vi "Target.vi"() -> ()   [LabVIEW 2018]
uses:
  <vilib>/Platform/TimedLoop/XDataNode/timing_clust.ctl
  <vilib>/Platform/TimedLoop/XDataNode/nitl_modes.ctl
  <vilib>/Platform/TimedLoop/XDataNode/wakeup.ctl
  <vilib>/rvi/eio/common/nirviEmuTemplateMethod_errors.vi
  <vilib>/rvi/Emulation/niFpgaSctlEmulationGetInTimedLoop.vi
  <vilib>/rvi/Emulation/niFpgaEmulationReportErrorSimple.vi
  <vilib>/rvi/Emulation/niFpgaGetClockAttributes.vi
  <vilib>/rvi/Emulation/niFpgaCriticalErrorInLSC.vi
  <vilib>/rvi/Emulation/niFpgaProcessEmulError.vi
  <vilib>/rvi/Memory/Memory_Emulation/niFpgaMemoryFastEmulationDramWriteAndRequestData.vi
  <vilib>/rvi/Memory/Memory_Emulation/niFpgaMemoryEmulationDramWriteAndRequestData.vi
  <vilib>/rvi/DataTransferAndStorage/Container/Common/niFpgaContainerGetUniqueNameForEmu.vi
  <vilib>/rvi/Memory/Memory_Emulation/niFpgaMemoryEmulationDramWriteAndRequestDataApplyByteEnables.vi
  <vilib>/rvi/interface/RandomDataEmulation/niFpgaRandomDataHandleErrors.vi
  <vilib>/eio/EIONode/EIONode.xnode
  <vilib>/Platform/TimedLoop/XDataNode/XDataNode.xnode
  <vilib>/rvi/DataTransferAndStorage/Container/XNode/niFpgaContainer.xnode
  <vilib>/rvi/Memory/Memory_Emulation/niFpgaMemoryEmulationDramRetrieveData.vi
  <vilib>/rvi/interface/RandomDataEmulation/nirviRandomDataFpgaReadWriteTemplate.vi
  <vilib>/Platform/TimedLoop/XDataNode/XDNodeRunTimeDep.lvlib
panel:
  in  "46":u8=46
  in  "94":u8=94
  in  "39":u8=39
  in  "95":u8=95
  in  "93":u8=93
  in  "38":u8=38
  in  "R35":u8=35
  in  "92":u8=92
  in  "75":u8=75
  in  "74":u8=74
  in  "56":u8=56
  in  "W35":u8=35
  in  "W75":u8=75
  in  "W1":u8=1
  in  "25":u8=25
  out "Read":bool[](array[boolean])
  in  "Write":bool[](array[boolean])=[FALSE, FALSE, FALSE, FALSE, FALSE, FALSE, FALSE, FALSE, FALSE, FALSE, FALSE, FALSE, FALSE, FALSE, FALSE, FALSE, FALSE, FALSE, FALSE, FALSE, FALSE, FALSE, FALSE, FALSE, FALSE, FALSE, FALSE, FALSE, FALSE, FALSE, FALSE, FALSE, FALSE, FALSE, FALSE]
  in  "Чтение_48":u8=48
  in  "Запись_38":u8=38
  in  "Запись(T)/Чтение(F)":bool
  in  "50":u8=50
  in  "EXPOSURE":bool
  in  "RESET_BAR":bool
  in  "STANDBY":bool
  in  "Кадр на ПК":bool
  in  "Нач_адр":u32
  in  "Кон_адр":u32=120320
  out "Записали FIFO":bool
  in  "Кадр в память":bool
  out "Записали адресов":u32
  in  "Направление бит":bool
  in  "360960":u32=360960
  in  "Стоп":bool
  in  "Регистр":bool
  # "Используется для записи и перед чтением"
  # "D0"
  # "D7"
  # "\"0\""
  # "D8"
  # "D15"
  # "\"0\""
  # "R0"
  # "R7"
  # "\"0\""
  # "А0"
  # "\"В8\" - запись"
  # "Режим \"Запись\""
  # "А7"
  # "А0"
  # "St"
  # "\"0\""
  # "R0"
  # "R7"
  # "\"0\""
  # "А0"
  # "\"В8\" - запись"
  # "А7"
  # "А7"
  # "\"В9\" - чтение"
  # "0"
  # "35"
  # "17 бит, поскольку ACK"
  # "0"
  # "16"
  # "7"
  # "8"
  # "ACK"
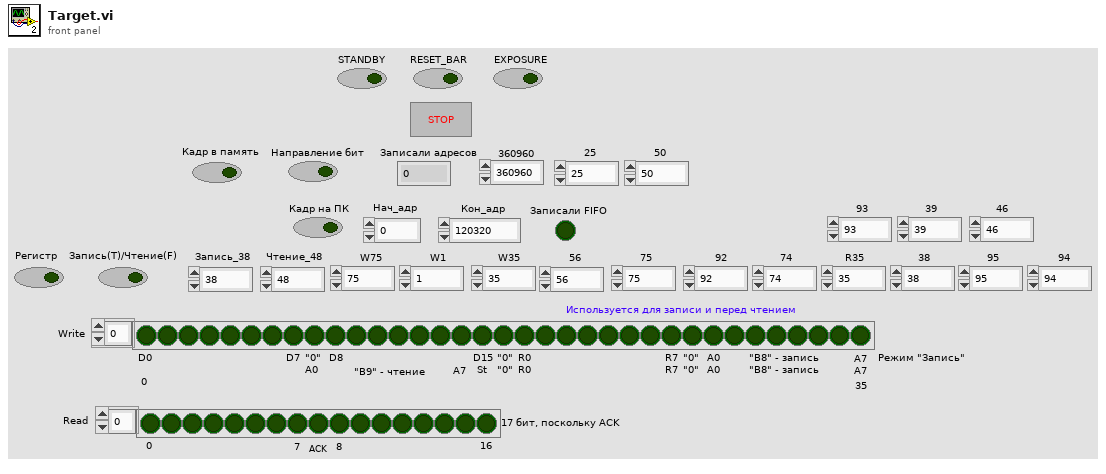
[diagram p1: front panel]
types:
  T1 = typedef "XDNodeRunTimeDep.lvlib/timing_clust.ctl" = cluster{"Expected End [f-1]":u64, "Actual End [f-1]":u64, "Finished Late? [f-1]":bool, "Expected End [i-1]":u64, "Actual End [i-1]":u64, "Finished Late? [i-1]":bool, "Expected Start [i]":u64, "Actual Start [i]":u64, "Expected Start [f]":u64, "Actual Start [f]":u64, "Source Name":string, "Structure Name":string, "Period":i64, "Deadline":i64, "Offset":i64, "Start":i64, "Priority":i32, "Timeout":i32, "Mode":T2, "Wakeup Reason":T3, "Error":errorcluster, "Source Type":string, "Secondary Source Type":string, "Global End Time":u64, "Global Start Time":u64, "Frame Duration":u64, "Iteration Duration":u64, "Assigned CPU":i32, "I/O Scan Engine Mode":u32}
  T2 = typedef "XDNodeRunTimeDep.lvlib/nitl_modes.ctl" = enum32{"No Change", "Process missed periods, maintain original phase", "Discard missed periods, maintain original phase", "Process missed periods, ignore original phase", "Discard missed periods, ignore original phase"}
  T3 = typedef "XDNodeRunTimeDep.lvlib/wakeup.ctl" = enum32{"Normal", "Aborted", "Asynchronous wakeup", "Timing source error", "Timed loop error", "Timeout"}
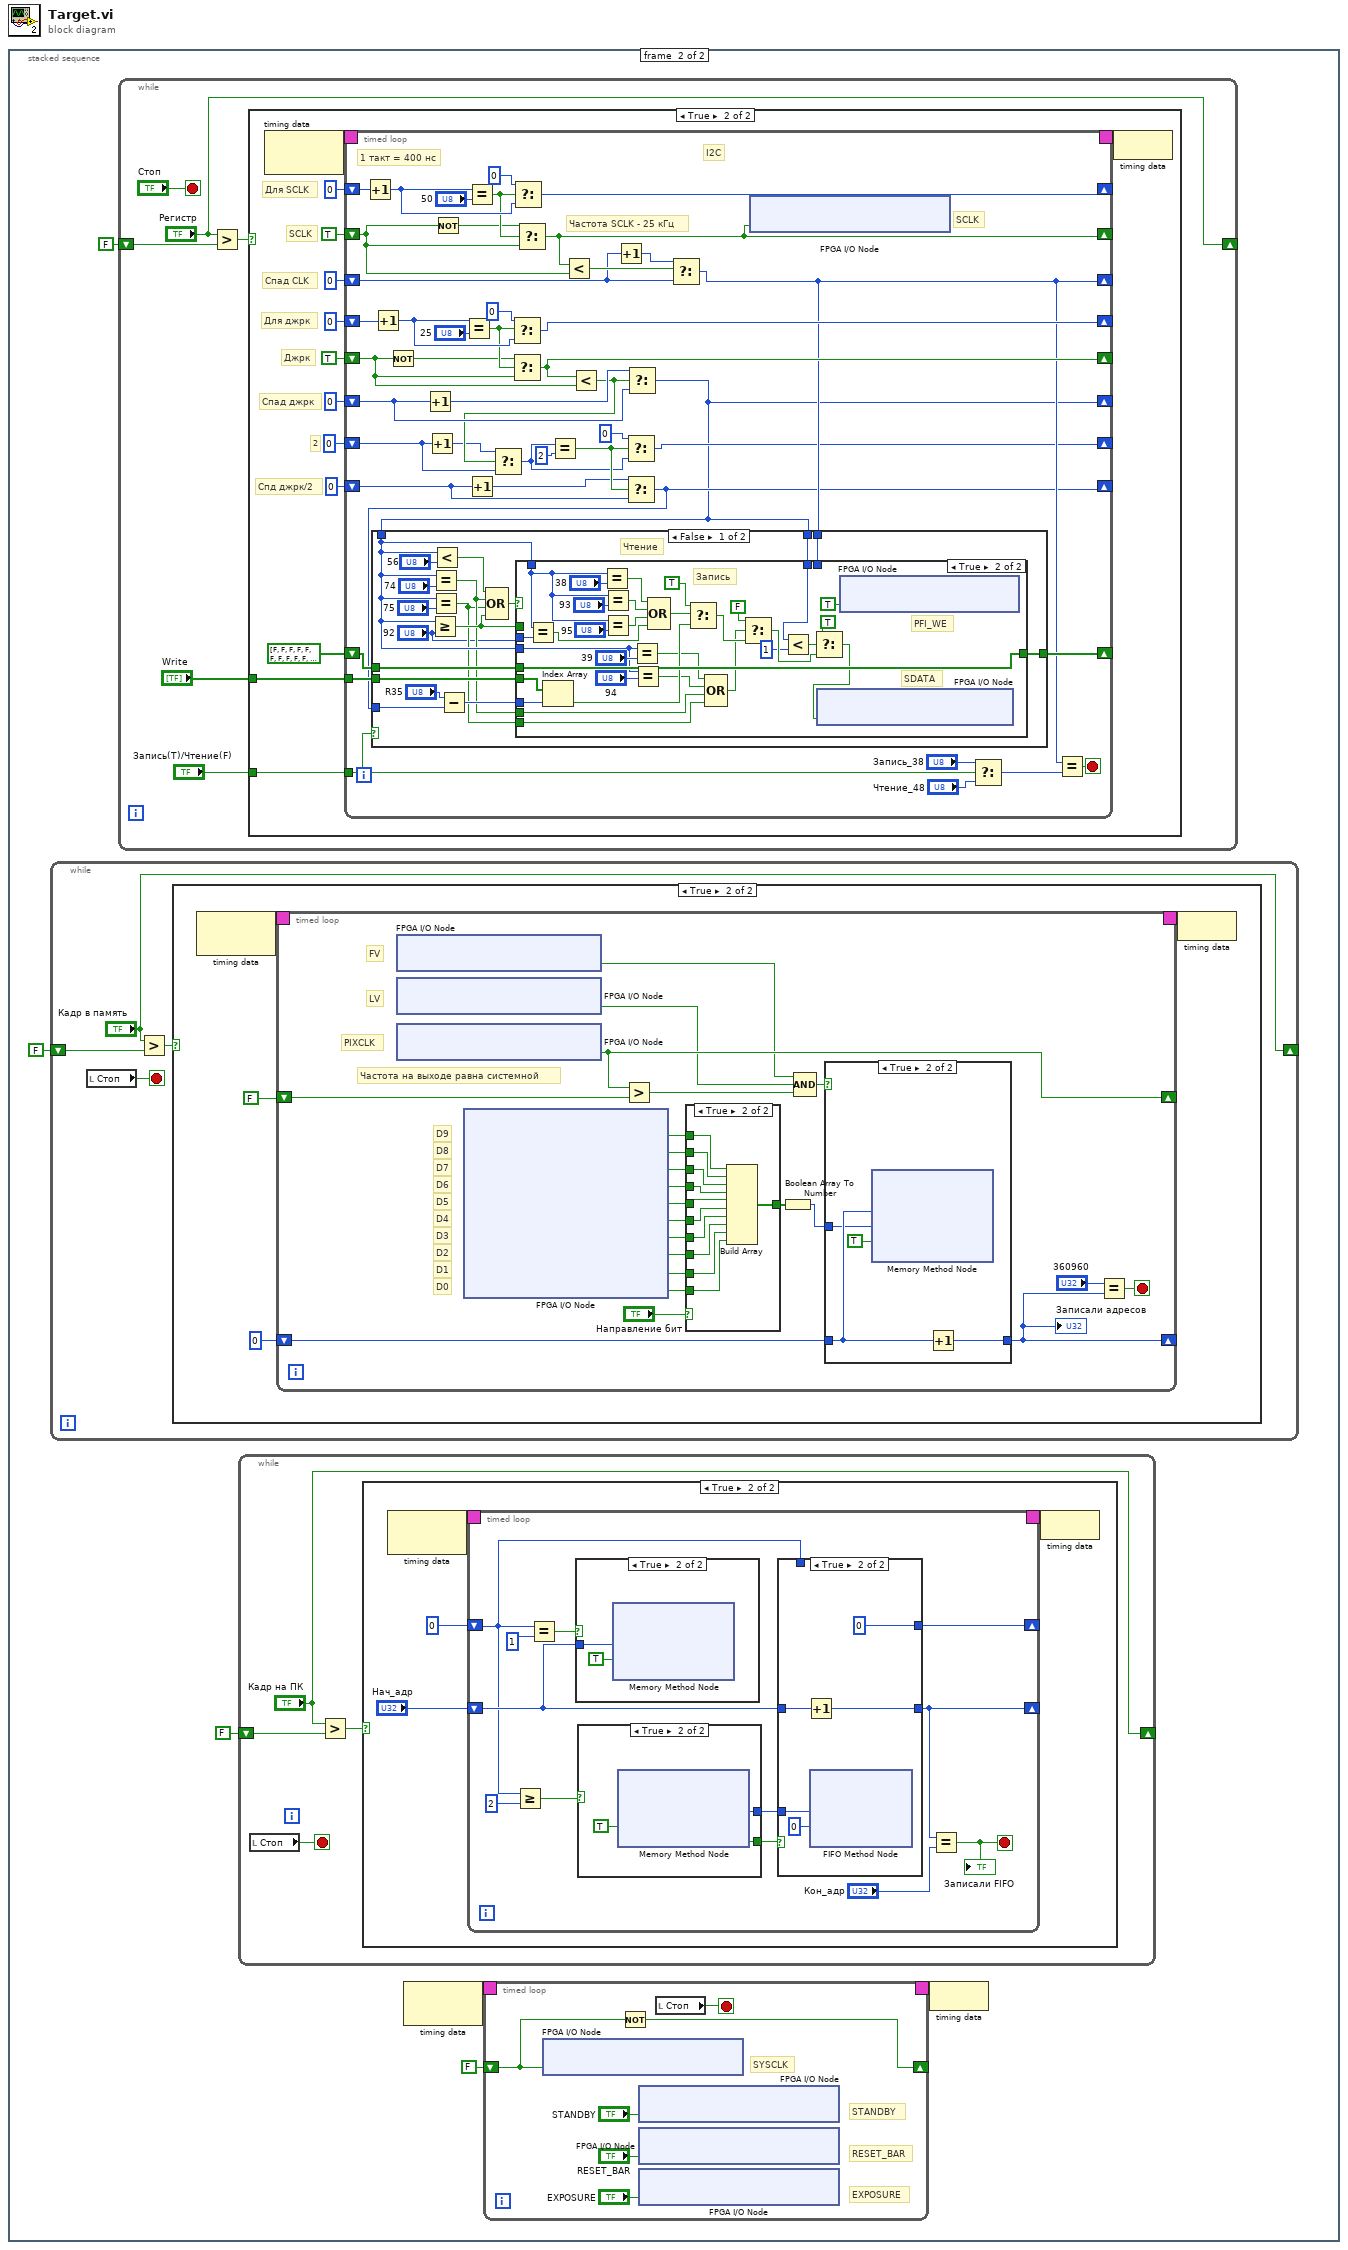
[diagram p0: block diagram]
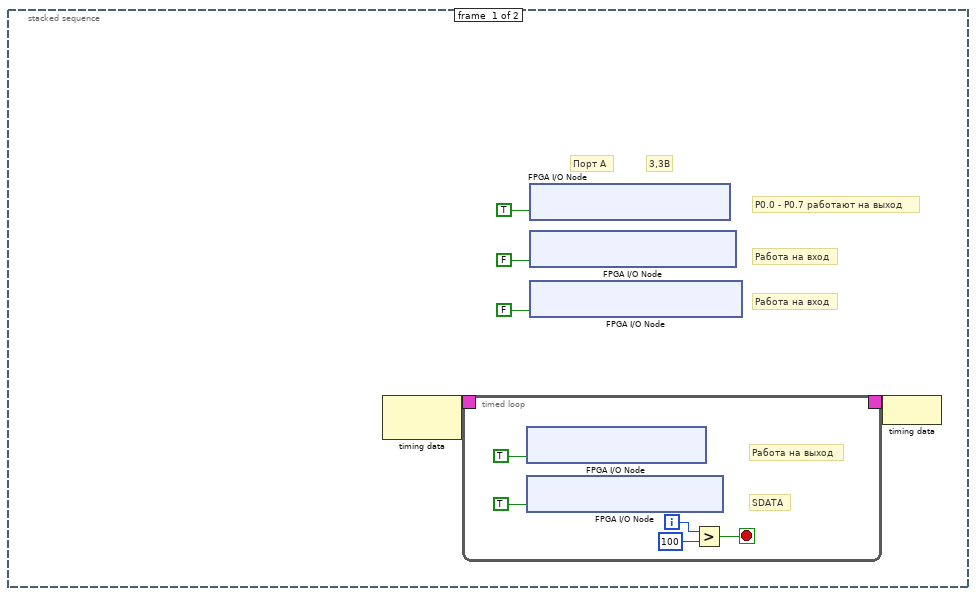
[diagram p2: hidden frame]
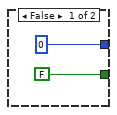
[diagram p4: hidden frame]
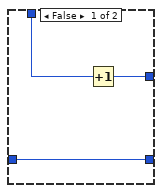
[diagram p6: hidden frame]
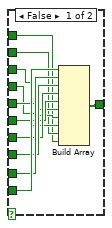
[diagram p8: hidden frame]
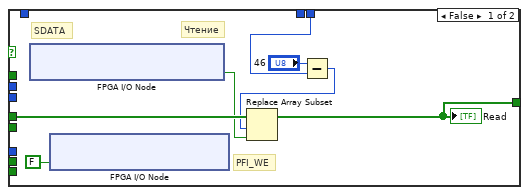
[diagram p11: hidden frame]
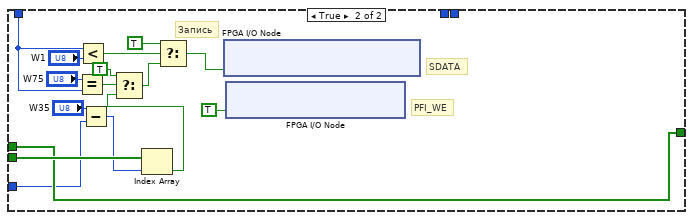
[diagram p12: hidden frame]
diagram:
  n1 = stacked-sequence {
    frame #0 {
      # "3,3В"
      # "Порт А"
      # "Работа на вход"
      # "Работа на вход"
      # "P0.0 - P0.7 работают на выход"
      n2 = node-c288() -> (w2:T1)  [unwired: 1 in]
      n3 = timed-loop {
        timing: w2 -> [_]
        timing-out: [_] -> w1
        i -> [w8]
        stop <- w6 stop-if-true
        # "SDATA"
        # "Работа на выход"
        n4 = xnode "FPGA I/O Node"("IO Module\\DDCA_PFI_WE"=TRUE ("IO Module\\DDCA_DIO16-23_WE")) -> ()  [unwired: 1 in, 1 out]
        n5 = xnode "FPGA I/O Node"("IO Module\\DDCA_PFI1_Write"=TRUE ("IO Module\\DDCA_PFI1_Write")) -> ()  [unwired: 1 in, 1 out]
        n6 = Greater?(x=w8, y=u8 100) -> (0:w6:bool)
      }
      n7 = xnode "FPGA I/O Node"("IO Module\\DDCA_DIO0-7_WE"=TRUE ("IO Module\\DDCA_DIO0-7_WE")) -> ()  [unwired: 1 in, 1 out]
      n8 = xnode "FPGA I/O Node"("IO Module\\DDCA_DIO8-15_WE"=FALSE ("IO Module\\DDCA_DIO8-15_WE")) -> ()  [unwired: 1 in, 1 out]
      n9 = xnode "FPGA I/O Node"("IO Module\\DDCA_DIO16-23_WE"=FALSE ("IO Module\\DDCA_DIO16-23_WE")) -> ()  [unwired: 1 in, 1 out]
      n10 = node-c288(w1) -> ()
    }
    frame #1 {
      n11 = while {
        shift-right: ["Кадр в память"] -> _
        shift-left: FALSE ("Кадр в память") -> [w72]
        stop <- w73 stop-if-true
        n12 = local read "Стоп"() -> (w73:bool)
        n13 = Greater?(x="Кадр в память", y=w72) -> (0:w71:bool)
        n14 = case shown="True" w71 {
          frame False {
          }
          frame True {
            n15 = node-c288() -> (w77:T1)  [unwired: 1 in]
            n16 = timed-loop {
              timing: w77 -> [_]
              timing-out: [_] -> w76
              shift-right: [w99] -> _
              shift-left: FALSE -> [w100]
              shift-right: [w86] -> _
              shift-left: u32 0 -> [w98]
              stop <- w84 stop-if-true
              # "Частота на выходе равна системной"
              # "D0"
              # "D1"
              # "PIXCLK"
              # "D2"
              # "D3"
              # "D4"
              # "D5"
              # "D6"
              # "D7"
              # "D8"
              # "D9"
              # "LV"
              # "FV"
              n17 = xnode "FPGA I/O Node"() -> ("IO Module\\DDCA_DIO20_Read"=w81:bool)  [unwired: 1 in, 1 out]
              n18 = xnode "FPGA I/O Node"() -> ("IO Module\\DDCA_DIO19_Read"=w78:bool)  [unwired: 1 in, 1 out]
              n19 = xnode "FPGA I/O Node"() -> ("IO Module\\DDCA_DIO12_Read"=w99:bool)  [unwired: 1 in, 1 out]
              n20 = xnode "FPGA I/O Node"() -> ("IO Module\\DDCA_DIO18_Read"=w96:bool, "IO Module\\DDCA_DIO21_Read"=w95:bool, "IO Module\\DDCA_DIO22_Read"=w94:bool, "IO Module\\DDCA_DIO23_Read"=w93:bool, "IO Module\\DDCA_DIO11_Read"=w92:bool, "IO Module\\DDCA_DIO16_Read"=w91:bool, "IO Module\\DDCA_DIO17_Read"=w90:bool, "IO Module\\DDCA_DIO15_Read"=w89:bool, "IO Module\\DDCA_DIO14_Read"=w83:bool, "IO Module\\DDCA_DIO13_Read"=w82:bool)  [unwired: 10 in, 10 out]
              n21 = Greater?(x=w99, y=w100) -> (0:w80:bool)
              n22 = case shown="True" "Направление бит" {
                tunnel: w96 -> [w101 w122]
                tunnel: w95 -> [w102 w121]
                tunnel: w94 -> [w103 w120]
                tunnel: w93 -> [w104 w119]
                tunnel: w92 -> [w105 w118]
                tunnel: w91 -> [w106 w117]
                tunnel: w90 -> [w107 w116]
                tunnel: w89 -> [w108 w115]
                tunnel: [w111 w114] -> w88
                tunnel: w83 -> [w109 w113]
                tunnel: w82 -> [w110 w112]
                frame False {
                  n23 = Build Array(w110, w109, w108, w107, w106, w105, w104, w103, w102, w101) -> (w111:bool[])
                }
                frame True {
                  n24 = Build Array(w122, w121, w120, w119, w118, w117, w116, w115, w113, w112) -> (w114:bool[])
                }
              }
              n25 = Boolean Array To Number(Boolean array=w88) -> (number=w87:u16)
              n26 = Compound Arithmetic op=AND(w81, w78, w80) -> (w79:bool)
              n27 = case shown="True" w79 {
                tunnel: w98 -> [w123 w127]
                tunnel: [w123 w126] -> w86
                tunnel: w87 -> [_ w125]
                frame False {
                }
                frame True {
                  n28 = xnode ("Memory Method Node")("Address"=w127, "Data"=w125, "Input Valid"=TRUE) -> ()  [unwired: 1 in, 2 out]
                  n29 = Increment(x=w127) -> (x+1=w126:u32)
                }
              }
              "Записали адресов" <- w86
              n30 = Equal?(x="360960", y=w86) -> (x = y?=w84:bool)
            }
            n31 = node-c288(w76) -> ()
          }
        }
      }
      n32 = while {
        shift-right: ["Регистр"] -> _
        shift-left: FALSE -> [w136]
        stop <- "Стоп" stop-if-true
        n33 = Greater?(x="Регистр", y=w136) -> (0:w137:bool)
        n34 = case shown="True" w137 {
          tunnel: "Запись(T)/Чтение(F)" -> [_ w145]
          tunnel: "Write" -> [_ w144]
          frame False {
          }
          frame True {
            # "2"
            # "Спд джрк/2"
            # "Спад джрк"
            # "Для джрк"
            # "SCLK"
            # "Для SCLK"
            # "Спад CLK"
            # "Джрк"
            n35 = node-c288() -> (w150:T1)  [unwired: 1 in]
            n36 = timed-loop {
              timing: w150 -> [_]
              timing-out: [_] -> w149
              shift-right: [w171] -> _
              shift-left: TRUE -> [w170]
              shift-right: [w190] -> _
              shift-left: u8 0 -> [w194]
              shift-right: [w185] -> _
              shift-left: TRUE -> [w184]
              tunnel: w145 -> [w167]
              tunnel: w144 -> [w166]
              shift-right: [w163] -> _
              shift-left: u8 0 -> [w182]
              shift-right: [w172] -> _
              shift-left: u8 0 -> [w178]
              shift-right: [w151] -> _
              shift-left: u8 0 -> [w168]
              shift-right: [w164] -> _
              shift-left: bool[] [FALSE, FALSE, FALSE, FALSE, FALSE, FALSE, FALSE, FALSE, FALSE, FALSE, FALSE, FALSE, FALSE, FALSE, FALSE, FALSE, FALSE] -> [w165]
              shift-right: [w158] -> _
              shift-left: u8 0 -> [w156]
              shift-right: [w160] -> _
              shift-left: u8 0 -> [w153]
              stop <- w179 stop-if-true
              # "1 такт = 400 нс"
              # "SCLK"
              # "Частота SCLK - 25 кГц"
              # "I2C"
              n37 = Increment(x=w194) -> (x+1=w192:u8)
              n38 = Increment(x=w178) -> (x+1=w175:u8)
              n39 = Not(x=w170) -> (.not. x?=w173:bool)
              n40 = Increment(x=w168) -> (x+1=w169:u8)
              n41 = Increment(x=w153) -> (x+1=w154:u8)
              n42 = Not(x=w184) -> (.not. x?=w188:bool)
              n43 = Equal?(x=w175, y="25") -> (x = y?=w174:bool)
              n44 = Equal?(x=w192, y="50") -> (x = y?=w189:bool)
              n45 = Increment(x=w156) -> (x+1=w157:u8)
              n46 = Select(t=u8 0, s=w174, f=w175) -> (s? t:f=w172:u8)
              n47 = Select(t=w173, s=w174, f=w170) -> (s? t:f=w171:bool)
              n48 = Select(t=u8 0, s=w189, f=w192) -> (s? t:f=w190:u8)
              n49 = Select(t=w188, s=w189, f=w184) -> (s? t:f=w185:bool)
              n50 = Less?(x=w185, y=w184) -> (x < y?=w183:bool)
              n51 = Less?(x=w171, y=w170) -> (x < y?=w155:bool)
              n52 = Select(t=w154, s=w155, f=w153) -> (s? t:f=w152:u8)
              n53 = Equal?(x=w152, y=u8 2) -> (x = y?=w159:bool)
              n54 = Increment(x=w182) -> (x+1=w181:u8)
              n55 = Select(t=u8 0, s=w159, f=w152) -> (s? t:f=w160:u8)
              n56 = Select(t=w157, s=w159, f=w156) -> (s? t:f=w158:u8)
              n57 = Select(t=w169, s=w155, f=w168) -> (s? t:f=w151:u8)
              n58 = Select(t=w181, s=w183, f=w182) -> (s? t:f=w163:u8)
              n59 = case shown="False" w167 {
                tunnel: w151 -> [w202 w260]
                tunnel: w166 -> [w205 w258]
                tunnel: w165 -> [w204 w254]
                tunnel: [w203 w254] -> w164
                tunnel: w163 -> [w201 _]
                tunnel: w158 -> [w196 w253]
                tunnel: w151 -> [w195 _]
                frame False {
                  # "Чтение"
                  n60 = Greater Or Equal?(x=w202, y="92") -> (x >= y?=w200:bool)
                  n61 = Equal?(x=w202, y="74") -> (x = y?=w199:bool)
                  n62 = Equal?(x=w202, y="75") -> (x = y?=w198:bool)
                  n63 = Less?(x=w202, y="56") -> (x < y?=w211:bool)
                  n64 = Subtract(x="R35", y=w196) -> (x-y=w206:u8)
                  n65 = Compound Arithmetic op=OR(w211, w199, w198, w200) -> (w208:bool)
                  n66 = case shown="True" w208 {
                    tunnel: w206 -> [_ w250]
                    tunnel: w205 -> [_ w249]
                    tunnel: w204 -> [w218 w248]
                    tunnel: [w217 w248] -> w203
                    tunnel: w202 -> [_ w227]
                    tunnel: w202 -> [_ w236]
                    tunnel: w201 -> [w214 _]
                    tunnel: w200 -> [_ _]
                    tunnel: w199 -> [_ w233]
                    tunnel: w198 -> [_ w230]
                    tunnel: "92" -> [_ w228]
                    tunnel: w195 -> [_ w224]
                    frame False {
                      # "SDATA"
                      # "PFI_WE"
                      # "Чтение"
                      n67 = xnode "FPGA I/O Node"() -> ("IO Module\\DDCA_PFI1_Read"=w216:bool)  [unwired: 1 in, 1 out]
                      n68 = xnode "FPGA I/O Node"("IO Module\\DDCA_PFI_WE"=FALSE ("IO Module\\DDCA_PFI_WE")) -> ()  [unwired: 1 in, 1 out]
                      n69 = Subtract(x="46", y=w214) -> (x-y=w213:u8)
                      n70 = Replace Array Subset(array=w218, new element=w216, index=w213) -> (w217:bool[])
                      "Read" <- w217
                    }
                    frame True {
                      # "SDATA"
                      # "PFI_WE"
                      # "Запись"
                      n71 = Equal?(x=w227, y=w228) -> (x = y?=w226:bool)
                      n72 = Index Array(array=w249, index=w250) -> (element=w241:bool)
                      n73 = Equal?(x=w227, y="38") -> (x = y?=w244:bool)
                      n74 = Equal?(x=w227, y="93") -> (x = y?=w235:bool)
                      n75 = Equal?(x=w227, y="95") -> (x = y?=w234:bool)
                      n76 = Equal?(x=w236, y="39") -> (x = y?=w232:bool)
                      n77 = Equal?(x=w236, y="94") -> (x = y?=w231:bool)
                      n78 = Compound Arithmetic op=OR(w244, w235, w234, w226) -> (w243:bool)
                      n79 = Select(t=TRUE, s=w243, f=w241) -> (s? t:f=w239:bool)
                      n80 = Compound Arithmetic op=OR(w232, w231, w233, w230) -> (w229:bool)
                      n81 = Select(t=FALSE, s=w229, f=w239) -> (s? t:f=w223:bool)
                      n82 = Less?(x=w224, y=u8 1 ("2WR")) -> (x < y?=w225:bool)
                      n83 = Select(t=TRUE, s=w225, f=w223) -> (s? t:f=w220:bool)
                      n84 = xnode "FPGA I/O Node"("IO Module\\DDCA_PFI1_Write"=w220) -> ()  [unwired: 1 in, 1 out]
                      n85 = xnode "FPGA I/O Node"("IO Module\\DDCA_PFI_WE"=TRUE ("IO Module\\DDCA_PFI_WE")) -> ()  [unwired: 1 in, 1 out]
                    }
                  }
                }
                frame True {
                  # "SDATA"
                  # "PFI_WE"
                  # "Запись"
                  n86 = Equal?(x="W75", y=w260) -> (x = y?=w264:bool)
                  n87 = Less?(x=w260, y="W1") -> (x < y?=w266:bool)
                  n88 = Subtract(x="W35", y=w253) -> (x-y=w257:u8)
                  n89 = Index Array(array=w258, index=w257) -> (element=w255:bool)
                  n90 = Select(t=TRUE, s=w264, f=w255) -> (s? t:f=w262:bool)
                  n91 = Select(t=TRUE, s=w266, f=w262) -> (s? t:f=w256:bool)
                  n92 = xnode "FPGA I/O Node"("IO Module\\DDCA_PFI1_Write"=w256) -> ()  [unwired: 1 in, 1 out]
                  n93 = xnode "FPGA I/O Node"("IO Module\\DDCA_PFI_WE"=TRUE ("IO Module\\DDCA_PFI_WE")) -> ()  [unwired: 1 in, 1 out]
                }
              }
              n94 = xnode "FPGA I/O Node"("IO Module\\DDCA_DIO6_Write"=w185) -> ()  [unwired: 1 in, 1 out]
              n95 = Select(t="Запись_38", s=w167, f="Чтение_48") -> (s? t:f=w180:u8)
              n96 = Equal?(x=w163, y=w180) -> (x = y?=w179:bool)
            }
            n97 = node-c288(w149) -> ()
          }
        }
      }
      n98 = while {
        shift-right: ["Кадр на ПК"] -> _
        shift-left: FALSE ("Кадр на ПК") -> [w32]
        stop <- w34 stop-if-true
        n99 = local read "Стоп"() -> (w34:bool)
        n100 = Greater?(x="Кадр на ПК", y=w32) -> (0:w33:bool)
        n101 = case shown="True" w33 {
          frame False {
          }
          frame True {
            n102 = node-c288() -> (w38:T1)  [unwired: 1 in]
            n103 = timed-loop {
              shift-right: [w49] -> _
              shift-left: "Нач_адр" -> [w43]
              timing: w38 -> [_]
              timing-out: [_] -> w37
              shift-right: [w40] -> _
              shift-left: u8 0 -> [w41]
              stop <- w50 stop-if-true
              n104 = Greater Or Equal?(x=w41, y=u8 2 ("2")) -> (x >= y?=w44:bool)
              n105 = Equal?(x=w41, y=u8 1 ("1")) -> (x = y?=w47:bool)
              n106 = case shown="True" w47 {
                tunnel: w43 -> [_ w56]
                frame False {
                }
                frame True {
                  n107 = xnode ("Memory Method Node")("Address"=w56, "Input Valid"=TRUE) -> ()  [unwired: 1 in, 2 out]
                }
              }
              n108 = case shown="True" w44 {
                tunnel: [u8 0 ("Data") w54] -> w48
                tunnel: [FALSE ("Output Valid") w53] -> w42
                frame False {
                }
                frame True {
                  n109 = xnode ("Memory Method Node")("Ready for Output"=TRUE ("Ready For Output")) -> ("Data"=w54:u16, "Output Valid"=w53:bool)  [unwired: 1 in, 1 out]
                }
              }
              n110 = case shown="True" w42 {
                tunnel: [w58 w65] -> w49
                tunnel: w48 -> [_ w61]
                tunnel: w43 -> [w58 w64]
                tunnel: w41 -> [w60 _]
                tunnel: [w59 u8 0] -> w40
                frame False {
                  n111 = Increment(x=w60) -> (x+1=w59:u8)
                }
                frame True {
                  n112 = Increment(x=w64) -> (x+1=w65:u32)
                  n113 = xnode ("FIFO Method Node")("Element"=w61, "Timeout"=0) -> ()  [unwired: 1 in, 2 out]
                }
              }
              n114 = Equal?(x=w49, y="Кон_адр") -> (x = y?=w50:bool)
              "Записали FIFO" <- w50
            }
            n115 = node-c288(w37) -> ()
          }
        }
      }
      n116 = node-c288() -> (w17:T1)  [unwired: 1 in]
      n117 = timed-loop {
        timing: w17 -> [_]
        timing-out: [_] -> w16
        shift-right: [w24] -> _
        shift-left: FALSE -> [w25]
        stop <- w26 stop-if-true
        # "EXPOSURE"
        # "RESET_BAR"
        # "STANDBY"
        # "SYSCLK"
        n118 = xnode "FPGA I/O Node"("IO Module\\DDCA_DIO0_Write"=w25) -> ()  [unwired: 1 in, 1 out]
        n119 = Not(x=w25) -> (.not. x?=w24:bool)
        n120 = xnode "FPGA I/O Node"("IO Module\\DDCA_DIO4_Write"="STANDBY") -> ()  [unwired: 1 in, 1 out]
        n121 = xnode "FPGA I/O Node"("IO Module\\DDCA_DIO5_Write"="RESET_BAR") -> ()  [unwired: 1 in, 1 out]
        n122 = xnode "FPGA I/O Node"("IO Module\\DDCA_DIO7_Write"="EXPOSURE") -> ()  [unwired: 1 in, 1 out]
        n123 = local read "Стоп"() -> (w26:bool)
      }
      n124 = node-c288(w16) -> ()
    }
  }
